vi "REFPROP1dll.vi"(8 "error in (no error)":errorcluster, 11 "Inputs":T2) -> (0 "error out":errorcluster, 3 "Outputs":T1)   [LabVIEW 2016]
doc: "subroutine REFPROP1dll(hIn, hOut, iUnits, iMass, a, b, z, c, q, ierr, herr, hIn_length, hOut_length,\nherr_length)\n\nShort version of subroutine REFPROP that eliminates the arrays and the need to send the fluid names each time.\n\nThe variable Output (which is an array) is not included here, rather the variable c returns the calculated value as\na double precision variable, and thus only one value can be returned at a time.\n\nIf the error number (ierr) is zero, the string contained in hUnits will be sent back in herr.\nAll other inputs and outputs are described in the REFPROPdll() vi.\n\nIf q (quality) returns a value between zero and one (and thus the state is two-phase), the REFPROP routine will\nbe needed to obtain the equilibrium compositions.\n\nINPUTS:\nhIn -- Input string of properties being sent to the routine.\nhOut -- Various flags are available to gain access to all other features of the REFPROP\nprogram.\niUnits -- The unit system to be used for the input and output properties (such as SI,\nEnglish, etc.) See the details much further below for a complete description of the iUnits\ninput value. NOTE: A mass based value for iUnits does not imply that the input and output\ncompositions are on a mass basis, this is specified with the iMass variable.\niMass -- Specifies if the input composition is mole or mass based\n0 Input compositions given in mole fractions, quality on a molar basis.\n1 Input compositions given in mass fractions, quality on a mass basis. For two-phase\nstates, the values in x and y will be returned on a mass basis if iMass=1. NOTE: If the\nfluid string sent to this routine contains the word “mass” at the end (and thus contains\nthe composition as well as the names of the fluids), this will have preference over the\nvalue of iMass when converting those compositions from a mass to a molar basis.\nHowever, compositions sent back will still be based on the value in iMass.\na -- First input property as specified in the hIn variable\nb -- Second input property as specified in the hIn variable\nz -- Composition on a mole or mass basis depending on the value sent in\niMass (array of size ncmax=20).\n\nOUTPUTS:\nc -- Output value. The number -9999970 will be returned when errors occur,\nand the number -9999990 will be returned when nothing was calculated. Read the comments\nin the ALLPROPS routine for more information.\nq -- Vapor quality on a mole or mass basis depending on the value of iMass.\n(See subroutine ABFLSH for the definitions of values returned for this variable). To obtain\nthe molar quality regardless of iMass, send “qmole” as an input in hIn, and vice-versa for\n“qmass”.\nierr -- Error flag\nherr -- Error string (character*255)\nhIn_length -- length of variable hIn (default: 255)\nhOut_length -- length of variable hOut (default: 255)\nherr_length -- length of variable herr (default: 255)"
uses:
  REFPROP.DLL
panel:
  # "REFPROP-REFPROP1dll.vi"
  # "void  REFPROP1dll(CStr hIn, CStr hOut, int32_t *iUnits, int32_t *iMass, double *a, double *b, double *z, double *c, double *q, int32_t *ierr, CStr herr, int32_t hIn_length, int32_t hOut_length, int32_t herr_length);"
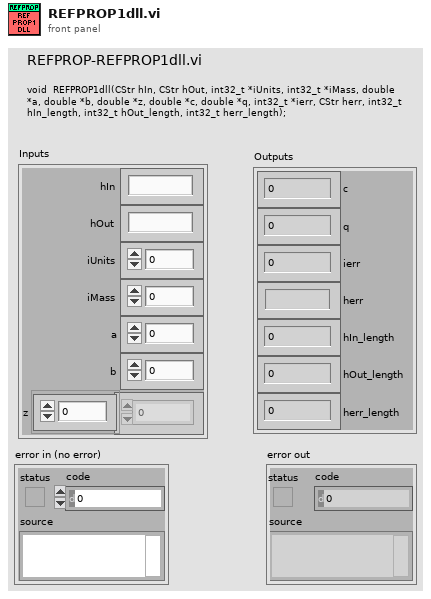
[diagram p1: front panel]
types:
  T1 = cluster{"c":dbl, "q":dbl, "ierr":i32, "herr":string, "hIn_length":i32, "hOut_length":i32, "herr_length":i32}
  T2 = cluster{"hIn":string, "hOut":string, "iUnits":i32, "iMass":i32, "a":dbl, "b":dbl, "z":dbl[]}
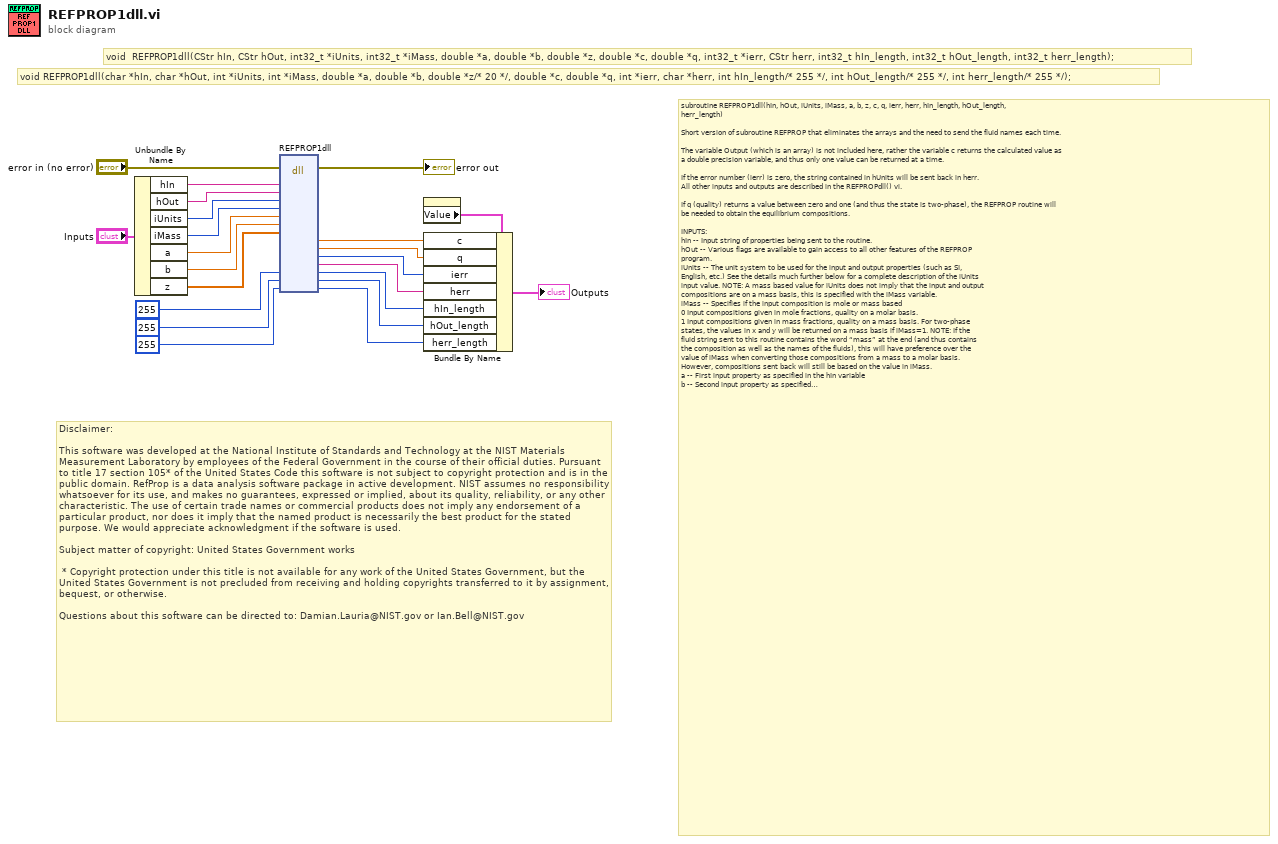
[diagram p0: block diagram]
diagram:
  # "void REFPROP1dll(char *hIn, char *hOut, int *iUnits, int *iMass, double *a, double *b, double *z/* 20 */, double *c, double *q, int *ierr, char *herr, int hIn_length/* 255 */, int hOut_length/* 255 */, int herr_length/* 255 */);"
  # "void  REFPROP1dll(CStr hIn, CStr hOut, int32_t *iUnits, int32_t *iMass, double *a, double *b, double *z, double *c, double *q, int32_t *ierr, CStr herr, int32_t hIn_length, int32_t hOut_length, int32_t herr_length);"
  # "subroutine REFPROP1dll(hIn, hOut, iUnits, iMass, a, b, z, c, q, ierr, herr, hIn_length, hOut_length,\nherr_length)\n\nShort version of subroutine REFPROP that eliminates the arrays and the need to send the fluid names each time.\n\nThe variable Output (which is an array) is not included here, rather the variable c returns the calculated value as\na double precision variable, and thus only one value can be returned at a time.\n\nIf the error number (ierr) is zero, the string contained in hUnits will be sent back in herr.\nAll other inputs and outputs are described in the REFPROPdll() vi.\n\nIf q (quality) returns a value between zero and one (and thus the state is two-phase), the REFPROP routine will\nbe needed to obtain the equilibrium compositions.\n\nINPUTS:\nhIn -- Input string of properties being sent to the routine.\nhOut -- Various flags are available to gain access to all other features of the REFPROP\nprogram.\niUnits -- The unit system to be used for the input and output properties (such as SI,\nEnglish, etc.) See the details much further below for a complete description of the iUnits\ninput value. NOTE: A mass based value for iUnits does not imply that the input and output\ncompositions are on a mass basis, this is specified with the iMass variable.\niMass -- Specifies if the input composition is mole or mass based\n0 Input compositions given in mole fractions, quality on a molar basis.\n1 Input compositions given in mass fractions, quality on a mass basis. For two-phase\nstates, the values in x and y will be returned on a mass basis if iMass=1. NOTE: If the\nfluid string sent to this routine contains the word “mass” at the end (and thus contains\nthe composition as well as the names of the fluids), this will have preference over the\nvalue of iMass when converting those compositions from a mass to a molar basis.\nHowever, compositions sent back will still be based on the value in iMass.\na -- First input property as specified in the hIn variable\nb -- Second input property as specified in the hIn variable\nz -- Composition on a mole or mass basis depending on the value sent in\niMass (array of size ncmax=20).\n\nOUTPUTS:\nc -- Output value. The number -9999970 will be returned when errors occur,\nand the number -9999990 will be returned when nothing was calculated. Read the comments\nin the ALLPROPS routine for more information.\nq -- Vapor quality on a mole or mass basis depending on the value of iMass.\n(See subroutine ABFLSH for the definitions of values returned for this variable). To obtain\nthe molar quality regardless of iMass, send “qmole” as an input in hIn, and vice-versa for\n“qmass”.\nierr -- Error flag\nherr -- Error string (character*255)\nhIn_length -- length of variable hIn (default: 255)\nhOut_length -- length of variable hOut (default: 255)\nherr_length -- length of variable herr (default: 255)"
  # "Disclaimer:\n\nThis software was developed at the National Institute of Standards and Technology at the NIST Materials Measurement Laboratory by employees of the Federal Government in the course of their official duties. Pursuant to title 17 section 105* of the United States Code this software is not subject to copyright protection and is in the public domain. RefProp is a data analysis software package in active development. NIST assumes no responsibility whatsoever for its use, and makes no guarantees, expressed or implied, about its quality, reliability, or any other characteristic. The use of certain trade names or commercial products does not imply any endorsement of a particular product, nor does it imply that the named product is necessarily the best product for the stated purpose. We would appreciate acknowledgment if the software is used.\n \nSubject matter of copyright: United States Government works\n  \n * Copyright protection under this title is not available for any work of the United States Government, but the United States Government is not precluded from receiving and holding copyrights transferred to it by assignment, bequest, or otherwise.\n\nQuestions about this software can be directed to: Damian.Lauria@NIST.gov or Ian.Bell@NIST.gov"
  n1 = Unbundle By Name("Inputs") -> ("hIn"=w13:string, "hOut"=w12:string, "iUnits"=w11:i32, "iMass"=w10:i32, "a"=w9:dbl, "b"=w8:dbl, "z"=w7:dbl[])
  n2 = dll-call lib="S:/009 - Testing/02 - Performance Testing/REFPROP/REFPROP.*" fn="REFPROP1dll"(error in="error in (no error)", "hIn"=w13, "hOut"=w12, "iUnits"=w11, "iMass"=w10, "a"=w9, "b"=w8, "z"=w7, "hIn_length"=255, "hOut_length"=255, "herr_length"=255) -> (error out=→"error out":errorcluster, "c"=w5:dbl, "q"=w19:dbl, "ierr"=w6:i32, "herr"=w18:string, "hIn_length"=w17:i32, "hOut_length"=w16:i32, "herr_length"=w15:i32)  [unwired: 14 in, 1 out]
  n3 = property on="Outputs" class="Clust (strict)"() -> ("Value"=w21:T1)  [unwired: 2 in, 2 out]
  n4 = Bundle By Name(cluster=w21, "c"=w5, "q"=w19, "ierr"=w6, "herr"=w18, "hIn_length"=w17, "hOut_length"=w16, "herr_length"=w15) -> (→"Outputs":T1)
